vi "Hybrid Stop Control Server.vi"(2 "error in (no error)":errorcluster, 3 "dup reference":refnum<vi>) -> (0 "error out":errorcluster)   [LabVIEW 2020]
doc: "This is a simple example of a server which exports VIs to be called from another machine. You may run both the client.llb and server.llb on the same machine without modifying the access list. If you wish to run the client on another machine that is not in your domain you will have to list the name of the client in the Machine Access List. \n\nThe VIs listed in the Exported VI list are exported by the server.\n\nTo run this example start this VI First, then start the client.llb on all machines you want to try as clients. If you change either of the above lists, you must restart this VI for the changes to take effect.\n\nClick the \"Stop\" button to quit. This will turn off the server, terminating all client connections, and restore the previous access lists to their original values."
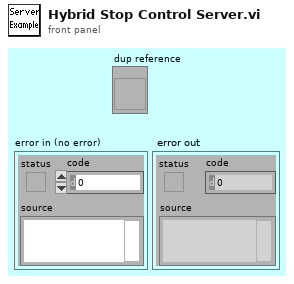
[diagram p1: front panel]
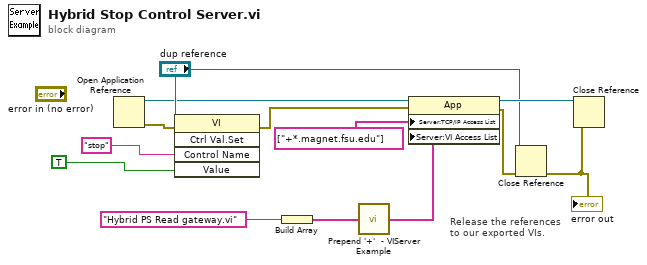
[diagram p0: block diagram]
diagram:
  # "Release the references\nto our exported VIs."
  n1 = Open Application Reference() -> (0:w9:errorcluster, 3:w7:refnum<vi>)  [unwired: 4 in]
  n2 = invoke class="VI" method="Ctrl Val.Set"(reference="dup reference", error in=w9, "Control Name"="stop", "Value"=TRUE) -> (error out=w6:errorcluster)  [unwired: 1 in, 4 out]
  n3 = Build Array("Hybrid PS Read gateway.vi") -> (w4:string[])
  n4 = call "Prepend '+'  - VIServer Example.vi"("list in"=w4) -> ("list out"=w2:string[])
  n5 = property class="App"(reference=w7, error in=w6, "Server:TCP/IP Access List"=string[] ["+*.magnet.fsu.edu"], "Server:VI Access List"=w2) -> (reference out=w13:refnum<vi>, error out=w12:errorcluster)
  n6 = Close Reference(reference="dup reference", error in (no error)=w12) -> (error out=w11:errorcluster)
  "error out" <- w11
  n7 = Close Reference(reference=w13, error in (no error)=w11) -> ()  [unwired: 1 out]
